vi "Loop.vi"(11 "Actor in":refnum<class "Actor.lvclass">) -> (3 "Actor out":refnum<class "Actor.lvclass">)   [LabVIEW 2021, in "Actor.lvclass"]
uses:
  Actor.lvclass
  Msg/Msg.lvclass
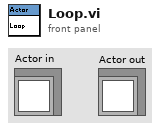
[diagram p1: front panel]
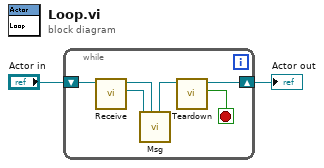
[diagram p0: block diagram]
diagram:
  n1 = while {
    shift-right: [w8] -> w1
    shift-left: "Actor in" -> [w5]
    stop <- w6 stop-if-true
    n2 = call-dynamic "Receive.vi"("Actor in"=w5) -> ("Msg"=w7:refnum<class "Msg.lvclass">, "Actor out"=w4:refnum<class "Actor.lvclass">)  [unwired: 9 in]
    n3 = call-dynamic "Msg.vi"("Actor in"=w4, "Msg in"=w7) -> ("Actor out"=w3:refnum<class "Actor.lvclass">)  [unwired: 9 in]
    n4 = call-dynamic "Teardown.vi"("Actor in"=w3) -> ("Teardown?"=w6:bool, "Actor out"=w8:refnum<class "Actor.lvclass">)  [unwired: 9 in]
  }
  "Actor out" <- w1
